vi "Reset_Instr.vi"(8 "error in (no error)":errorcluster caption="entrée d'erreur (pas d'erreur)", 11 "Class Relay_Board en entrée":refnum<class "Class Instrument Relay_Board.lvclass">) -> (0 "error out":errorcluster caption="sortie d'erreur", 3 "Class Relay_Board en Sortie":refnum<class "Class Instrument Relay_Board.lvclass">)   [LabVIEW 2020, in "Library Instrument & Equipement.lvlib" / "Library Instruments.lvlib" / "Class Instrument Relay_Board.lvclass"]
uses:
  Class Instrument Relay_Board.lvclass
  Class Instrument Relay_Board.lvclass/Class Instrument Relay_Board.ctl
  Instrument (Default)/Class Instrument (Default).lvclass
  Relay_Board/Relay_Board (Default)/Class Relay_Board (Default).lvclass
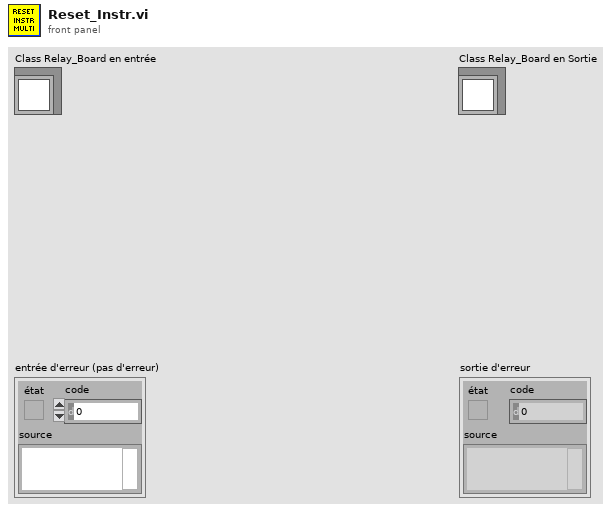
[diagram p1: front panel]
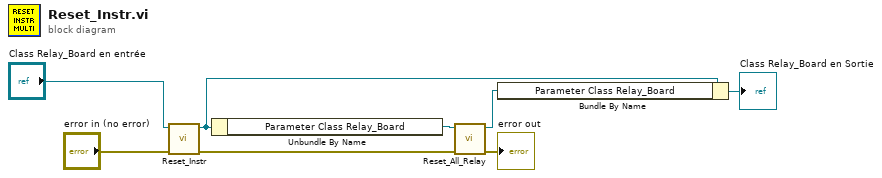
[diagram p0: block diagram]
diagram:
  n1 = call-parent "Reset_Instr.vi"("error in (no error)"="error in (no error)", "Class Instrument (Default) en entrée"="Class Relay_Board en entrée") -> ("error out"=w6:errorcluster, "Class Instrument (Default) en sortie"=w1:refnum<class "Class Instrument Relay_Board.lvclass">)  [unwired: 8 in]
  n2 = Unbundle By Name(w1) -> ("Parameter Class Relay_Board"=w4:refnum<class "Class Relay_Board (Default).lvclass">)
  n3 = call-dynamic "Reset_All_Relay.vi"("error in (no error)"=w6, "Class Relay_Board (Default) en entrée"=w4) -> ("error out"=→"error out":errorcluster, "Class Relay_Board (Default) en sortie"=w2:refnum<class "Class Relay_Board (Default).lvclass">)  [unwired: 8 in]
  n4 = Bundle By Name(cluster=w1, "Parameter Class Relay_Board"=w2) -> (→"Class Relay_Board en Sortie":refnum<class "Class Instrument Relay_Board.lvclass">)
